vi "SV Multitone SINAD and THD+N (Time) (1 Ch).vi"(0 "response signal [EU]":waveform(dbl), 1 "reference tones":T1(array[cluster]) {"phase (deg)" format="%0.3p"; "amplitude [EU pk]" format="%0.3p"; "frequency [Hz]" format="%0.3p"}, 2 "frequency range":T12={"start frequency"=-1.0, "stop frequency"=-1.0} {"stop frequency" format="%.2f"; "start frequency" format="%.2f"}, 3 "advanced span [Hz]":dbl=-1.0 format="%.2f", 5 "error in (no error)":errorcluster, 6 "desired units":T2={"SINAD"=enum."dB", "THD+N"=enum."dB", "response level"=enum."EU rms", "noise and distortion level"=enum."EU rms"}) -> (12 "unit labels":T3, 14 "complex spectrum response":T10={"complex spectrum response"={"f0"=0.0, "df"=1.0, "complex spectrum"=[]}, "spectrum info"={"channel name"="", "description"="", "x-axis units"=0, "spectral info"={"spectrum type"=enum."Power [Magnitude^2]", "linear/dB"=enum."linear", "window"=0, "window size"=0, "FFT size"=0}, "engineering units"=0, "custom label"="", "dB reference [EU]"=0.0, "peak units"=enum."rms", "weighting filter"=0, "spectral density?"=FALSE, "unit label"="", "spectrum skewed?"=FALSE, "complimentary spectrum units"=enum."none"}} {"spectrum info"."x-axis units" items=["Time (s)"=0, "Frequency-CB (Hz)"=1, "Frequency-CPB (Hz)"=1248, "Frequency-Arbitrary (Hz)"=2357, "Quefrency (s)"=2, "Revolutions (rev)"=3, "Order"=4, "Speed (RPM)"=11, "Speed (rad/s)"=21, "Index"=65535]; "spectrum info"."weighting filter" items=["Linear", "A-weighting", "B-weighting", "C-weighting", "ITU-R 468-4", "Dolby", "CCITT", "C-message", "Wb", "Wc", "Wd", "We", "Wf", "Wh", "Wj", "Wk", "Wm", "AES17 20 kHz lowpass", "AES17 40 kHz lowpass", "AES17 20 kHz highpass", "AES17 40 kHz highpass"]; "spectrum info"."dB reference [EU]" format="%.2f"; "spectrum info"."engineering units" items=["custom..."=0, "V"=1, "A"=21, "C"=30, "pC"=31, "s"=32, "-"=29, "Pa"=2, "N"=20, "g"=3, "m/s^2"=4, "m/s"=5, "m"=6, "mm/s"=12, "mm"=13, "micron/s"=14, "micron"=15, "in/s^2"=7, "in/s"=8, "in"=9, "mil/s"=10, "mil"=11, "rad/s^2"=16, "rad/s"=17, "rad"=18, "deg/s^2"=26, "deg/s"=27, "deg"=28, "RPM"=22, "cycle/s^2"=23, "Hz"=24, "cycle"=25, "strain"=19]; "spectrum info"."spectral info"."window" items=["None "=0, "Hanning"=1, "Hamming"=2, "Blackman-Harris"=3, "Exact Blackman"=4, "Blackman"=5, "Flat Top"=6, "4 Term B-Harris "=7, "7 Term B-Harris"=8, "Low Sidelobe"=9, "Force - Exponential"=10, "Gaussian"=62]; "complex spectrum response"."complex spectrum" format="%.2f"; "complex spectrum response"."df" format="%.2f"; "complex spectrum response"."f0" format="%.2f"}, 15 "SINAD":dbl format="%.2f", 16 "THD+N":dbl format="%.2f", 18 "levels":T11 {"noise and distortion" format="%.2f"; "response" format="%.2f"}, 19 "error out":errorcluster)   [LabVIEW 2017, in "SoundVib_Multitone.lvlib"]
doc: "Performs a signal in noise and distortion (SINAD) analysis and analyzes total harmonic distortion plus noise (THD + N), including measuring the fundamental tones, and returns the and SINAD and THD + N in the desired units. Wire data to the <B>scaled signal [EU]</B> input to determine the polymorphic instance to use or manually select the instance.\n\nThe following formula calculates SINAD:\n\nSINAD = sqrt(F2 + N2 + H2) / sqrt(H2 + N2)\n\nwhere F is the fundamental tone RMS level, N is the noise RMS level, and H is the harmonic RMS level."
uses:
  <vilib>/addons/Sound and Vibration/svt_Multitone Distortion/SoundVib_Multitone.lvlib
  <vilib>/addons/_NISVFA/_Shared subVIs/Controls/svc_Spectrum Info.ctl
  <vilib>/addons/_NISVFA/_Shared subVIs/Controls/svc_X-Axis Units.ctl
  <vilib>/addons/_NISVFA/_Shared subVIs/Controls/svc_Spectrum Type.ctl
  <vilib>/addons/_NISVFA/_Shared subVIs/Controls/svc_Engineering Units Text Ring.ctl
  <vilib>/addons/_NISVFA/_Shared subVIs/Controls/svc_Weighting Filter Text Ring.ctl
  <vilib>/addons/_NISVFA/_Shared subVIs/Controls/svc_Complimentary Spectrum Units.ctl
  <vilib>/addons/_NISVFA/_Shared subVIs/Controls/svc_Window.ctl
  <vilib>/addons/Sound and Vibration/svt_Distortion/SoundVib_Distortion.lvlib
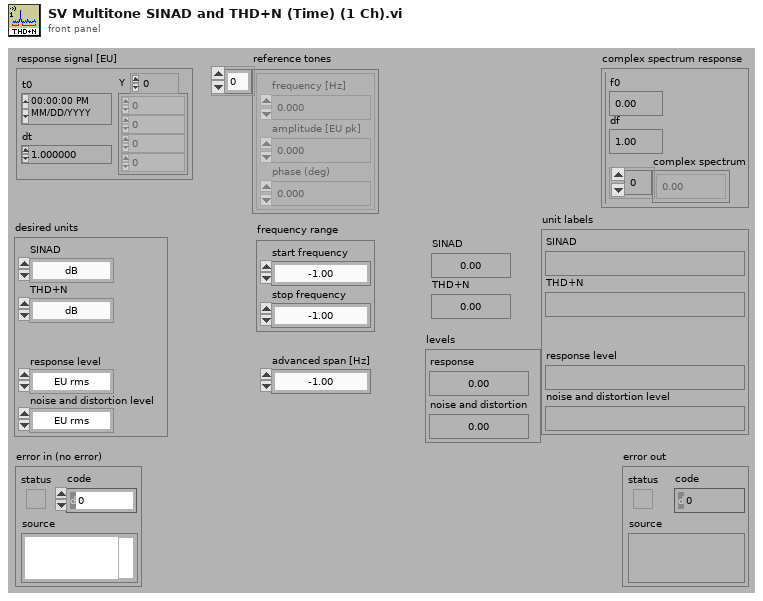
[diagram p1: front panel]
types:
  T1 = cluster{"frequency [Hz]":dbl, "amplitude [EU pk]":dbl, "phase (deg)":dbl}[]
  T2 = cluster{"SINAD":enum16{"dB", "linear ratio", "%"}, "THD+N":enum16{"dB", "linear ratio", "%"}, "response level":enum16{"EU^2 rms", "EU rms", "dB", "dBc", "dBV", "dBu", "dBm"}, "noise and distortion level":enum16{"EU^2 rms", "EU rms", "dB", "dBc", "dBV", "dBu", "dBm"}}
  T3 = cluster{"SINAD":string, "THD+N":string, "response level":string, "noise and distortion level":string}
  T4 = typedef "svc_Spectrum Info.ctl" = cluster{"channel name":string, "description":string, "x-axis units":T5, "spectral info":cluster{"spectrum type":T6, "linear/dB":enum16{"linear", "dB"}, "window":u16, "window size":i32, "FFT size":i32}, "engineering units":T7, "custom label":string, "dB reference [EU]":dbl, "peak units":enum16{"rms", "peak", "peak-peak"}, "weighting filter":T8, "spectral density?":bool, "unit label":string, "spectrum skewed?":bool, "complimentary spectrum units":T9}
  T5 = typedef "svc_X-Axis Units.ctl" = u16
  T6 = typedef "svc_Spectrum Type.ctl" = enum16{"FFT Spectrum [complex]", "Amplitude [Magnitude]", "Power [Magnitude^2]", "Cross Spectrum [complex]", "Frequency Response [Complex]"}
  T7 = typedef "svc_Engineering Units Text Ring.ctl" = u16
  T8 = typedef "svc_Weighting Filter Text Ring.ctl" = u16
  T9 = typedef "svc_Complimentary Spectrum Units.ctl" = enum16{"none", "radians", "degrees", "cycles", "imaginary"}
  T10 = cluster{"complex spectrum response":cluster{"f0":dbl, "df":dbl, "complex spectrum":cdb[]}, "spectrum info":T4}
  T11 = cluster{"response":dbl, "noise and distortion":dbl}
  T12 = cluster{"start frequency":dbl, "stop frequency":dbl}
  T13 = typedef "svc_Window.ctl" = u32
  T14 = cluster{"complex spectrum":cluster{"f0":dbl, "df":dbl, "complex spectrum":cdb[]}, "spectrum info":T4}
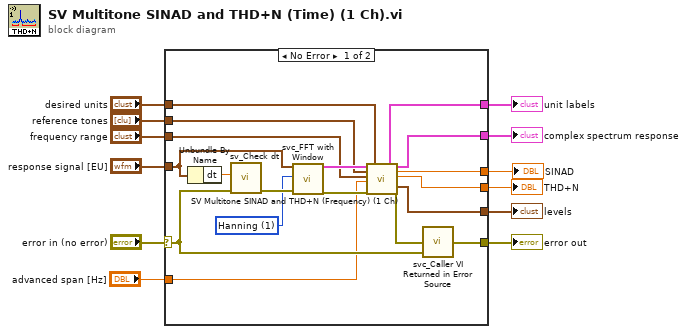
[diagram p0: block diagram]
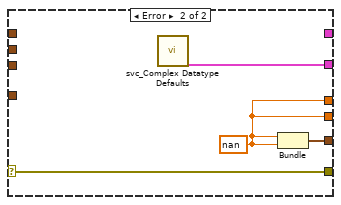
[diagram p2: hidden frame]
diagram:
  n1 = case shown="No Error" "error in (no error)" {
    selector: "error in (no error)" -> [w18 w34]
    tunnel: "response signal [EU]" -> [w20 _]
    tunnel: [w23 w34] -> w11
    tunnel: [w14 w32] -> w10
    tunnel: [w28 _] -> w8
    tunnel: [w27 w33] -> w7
    tunnel: "frequency range" -> [w26 _]
    tunnel: "desired units" -> [w25 _]
    tunnel: [w15 w32] -> w4
    tunnel: "reference tones" -> [w17 _]
    tunnel: "advanced span [Hz]" -> [w16 _]
    tunnel: [w13 w31] -> w1
    frame No Error {
      w21 = T13 1 items=["None ", "Hanning", "Hamming", "Blackman-Harris", "Exact Blackman", "Blackman", "Flat Top", "4 Term B-Harris ", "7 Term B-Harris", "Low Sidelobe", "Force - Exponential", "Gaussian"] ("window")
      n2 = Unbundle By Name(w20) -> ("dt"=w19:dbl)
      n3 = call <vilib>:"sv_Check dt.vi"("error in"=w18, "dt"=w19) -> ("error out"=w22:errorcluster)  [unwired: 8 in, 1 out]
      n4 = call <vilib>:"svc_FFT with Window.vi"("time signal in [EU]"=w20, "window"=w21, "error in (no error)"=w22) -> ("complex spectrum"=w30:T10, "error out"=w29:errorcluster)  [unwired: 15 in]
      n5 = call <vilib>:"SV Multitone SINAD and THD+N (Frequency) (1 Ch).vi"("complex spectrum response"=w30, "reference tones"=w17, "frequency range"=w26, "advanced span [Hz]"=w16, "error in (no error)"=w29, "desired units"=w25) -> ("unit labels"=w28:T3, "complex spectrum response"=w27:T10, "SINAD"=w15:dbl, "THD+N"=w14:dbl, "levels"=w13:T11, "error out"=w24:errorcluster)  [unwired: 8 in]
      n6 = call <vilib>:"svc_Caller VI Returned in Error Source.vi"("warning input to caller"=w18, "error in (no error)"=w24) -> ("error out"=w23:errorcluster)  [unwired: 3 in]
    }
    frame Error {
      w32 = nan ("SINAD")
      n7 = call <vilib>:"svc_Complex Datatype Defaults.vi"() -> ("complex spectrum"=w33:T14)  [unwired: 11 in, 8 out]
      n8 = Bundle("SINAD"=w32, "SINAD"=w32) -> (w31:cluster{"SINAD":dbl, "SINAD":dbl})  [unwired: 1 in]
    }
  }
  "error out" <- w11
  "THD+N" <- w10
  "levels" <- w1
  "complex spectrum response" <- w7
  "unit labels" <- w8
  "SINAD" <- w4
